vi "Send command (standalone).vi"(3 "Value":u16, 4 "Command":T2=17 items=["Measured main TEC temperature"=0, "Measured SHG heater temperature"=1, "Measured BRF heater temperature"=2, "Main TEC temperature command"=3, "SHG heater temperature command"=4, "BRF heater temperature command"=5, "Main TEC drive"=6, "SHG heater drive"=7, "BRF heater drive"=8, "Output power from photodiode"=9, "Output power setpoint (Get)"=10, "Output power setpoint (Set)"=11, "Start-up power setting (Get)"=12, "Start-up power setting (Set)"=13, "Measured LDD current"=14, "Maximum LDD current limit"=15, "16-bit fault code"=16, "Head serial number"=17, "Head board rev"=18, "Head type"=19, "LDD enable state"=20, "Key switch command (Get)"=24, "Key switch command (Set)"=25, "Key switch actual"=26, "Interlock status"=27, "Head hours"=28, "Photo or current mode command (Get)"=29, "Photo or current mode command (Set)"=30, "Photo or current mode actual"=31, "Analog input enable command (Get)"=32, "Analog input enable command (Set)"=33, "Analog input actual"=34, "Power supply glue input"=36, "Power supply glue output"=37], 5 "Selected laser":T1 items=["Green Laser", "Blue Laser"]) -> (0 "Error":errorcluster, 1 "response value":sgl, 2 "response":string)   [LabVIEW 2014]
uses:
  Commands.ctl
  Laser enum.ctl
  Coherent global.vi
panel:
  # "PN 06/11/2014"
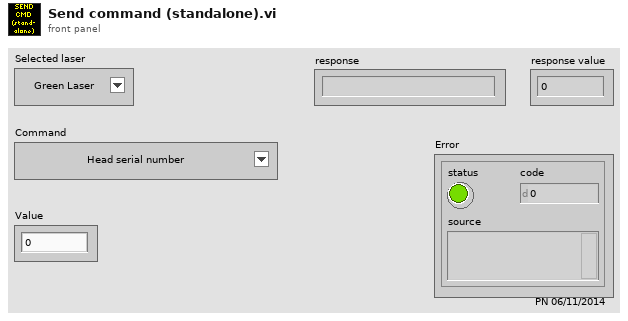
[diagram p1: front panel]
types:
  T1 = typedef "Laser enum.ctl" = u8
  T2 = typedef "Commands.ctl" = u8
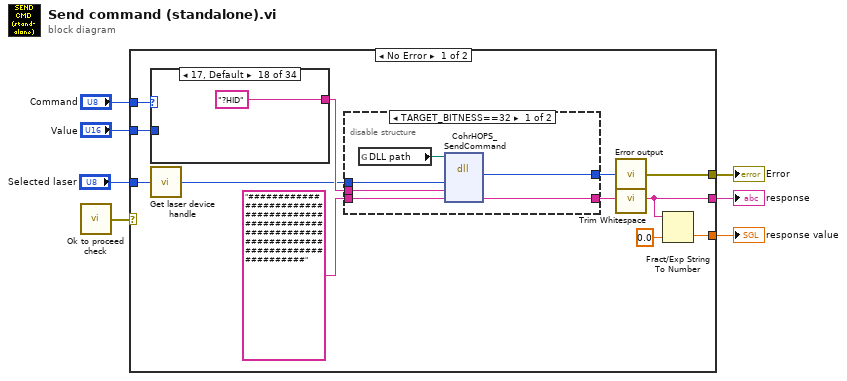
[diagram p0: block diagram]
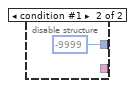
[diagram p2: hidden frame]
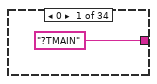
[diagram p3: hidden frame]
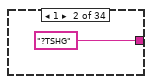
[diagram p4: hidden frame]
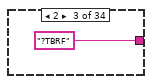
[diagram p5: hidden frame]
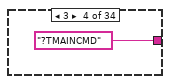
[diagram p6: hidden frame]
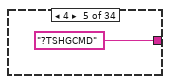
[diagram p7: hidden frame]
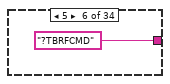
[diagram p8: hidden frame]
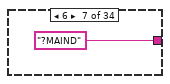
[diagram p9: hidden frame]
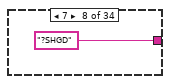
[diagram p10: hidden frame]
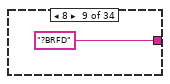
[diagram p11: hidden frame]
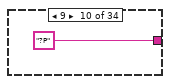
[diagram p12: hidden frame]
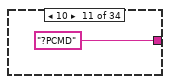
[diagram p13: hidden frame]
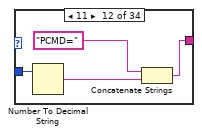
[diagram p14: hidden frame]
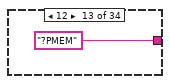
[diagram p15: hidden frame]
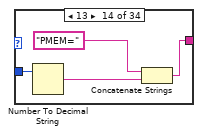
[diagram p16: hidden frame]
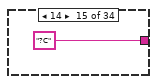
[diagram p17: hidden frame]
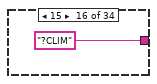
[diagram p18: hidden frame]
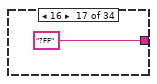
[diagram p19: hidden frame]
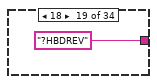
[diagram p20: hidden frame]
diagram:
  n1 = call "Ok to proceed check.vi"() -> ("Error"=w7:errorcluster)
  n2 = case shown="No Error" w7 {
    selector: w7 -> [_ w78]
    tunnel: [w14 sgl 0.0] -> w6
    tunnel: [w13 "" ("trimmed string")] -> w5
    tunnel: [w12 w78] -> w4
    tunnel: "Command" -> [w11 _]
    tunnel: "Value" -> [w10 _]
    tunnel: "Selected laser" -> [w9 _]
    frame No Error {
      n3 = case shown="17, Default" w11 {
        tunnel: ["?TMAIN" "?TSHG" "?TBRF" "?TMAINCMD" "?TSHGCMD" "?TBRFCMD" "?MAIND" "?SHGD" "?BRFD" "?P" "?PCMD" w38 "?PMEM" w43 "?C" "?CLIM" "?FF" "?HID" "?HBDREV" "?HTYPE" "?L" "?KSWCMD" w56 "?KSW" "?INT" "?HH" "?CMODECMD" w64 "?CMODE" "?ANACMD" w70 "?ANA" "?PSGLUEIN" "?PSGLUEOUT"] -> w18
        tunnel: w10 -> [_ _ _ _ _ _ _ _ _ _ _ w41 _ w46 _ _ _ _ _ _ _ _ w58 _ _ _ _ w66 _ _ w72 _ _ _]
        frame 0 {
        }
        frame 1 {
        }
        frame 2 {
        }
        frame 3 {
        }
        frame 4 {
        }
        frame 5 {
        }
        frame 6 {
        }
        frame 7 {
        }
        frame 8 {
        }
        frame 9 {
        }
        frame 10 {
        }
        frame 11 {
          n4 = Number To Decimal String(number=w41) -> (decimal integer string=w40:string)  [unwired: 1 in]
          n5 = Concatenate Strings("PCMD=", w40) -> (w38:string)
        }
        frame 12 {
        }
        frame 13 {
          n6 = Number To Decimal String(number=w46) -> (decimal integer string=w45:string)  [unwired: 1 in]
          n7 = Concatenate Strings("PMEM=", w45) -> (w43:string)
        }
        frame 14 {
        }
        frame 15 {
        }
        frame 16 {
        }
        frame 17, Default {
        }
        frame 18 {
        }
        frame 19 {
        }
        frame 20 {
        }
        frame 24 {
        }
        frame 25 {
          n8 = Number To Decimal String(number=w58) -> (decimal integer string=w55:string)  [unwired: 1 in]
          n9 = Concatenate Strings("KSWCMD=", w55) -> (w56:string)
        }
        frame 26 {
        }
        frame 27 {
        }
        frame 28 {
        }
        frame 29 {
        }
        frame 30 {
          n10 = Number To Decimal String(number=w66) -> (decimal integer string=w63:string)  [unwired: 1 in]
          n11 = Concatenate Strings("CMODECMD=", w63) -> (w64:string)
        }
        frame 31 {
        }
        frame 32 {
        }
        frame 33 {
          n12 = Number To Decimal String(number=w72) -> (decimal integer string=w69:string)  [unwired: 1 in]
          n13 = Concatenate Strings("ANACMD=", w69) -> (w70:string)
        }
        frame 34 {
        }
        frame 36 {
        }
        frame 37 {
        }
      }
      n14 = call "Get laser device handle.vi"("Selected laser"=w9) -> ("Device handle"=w8:u32)
      n15 = disable-structure shown="TARGET_BITNESS==32" {
        disable-tunnel: "####################################################################################################" ("headType") -> [w25 _]
        disable-tunnel: w8 -> [w24 _]
        disable-tunnel: w18 -> [w23 _]
        disable-tunnel: [w22 -9999 ("return value")] -> w17
        disable-tunnel: [w21 _] -> w16
        frame condition #0 (active) {
          n16 = global read "Coherent global.vi" "DLL path"() -> (w20:path)
          n17 = dll-call lib="C:/Program Files (x86)/Coherent/HOPS/CohrHOPS.dll" fn="CohrHOPS_SendCommand"(path in=w20, "handle"=w24, "command"=w23, "response"=w25) -> ("return value"=w22:i32, "response"=w21:string)  [unwired: 4 in, 2 out]
        }
        frame condition #1 {
        }
      }
      n18 = call "Error output.vi"("I32 err code"=w17) -> ("Error Out"=w12:errorcluster)
      n19 = call <vilib>:"Trim Whitespace.vi"("string"=w16) -> ("trimmed string"=w13:string)  [unwired: 1 in]
      n20 = Fract/Exp String To Number(string=w13, default (0 dbl)=sgl 0.0 ("default (0 DBL)")) -> (number=w14:sgl)  [unwired: 2 in, 1 out]
    }
    frame Error {
    }
  }
  "response" <- w5
  "response value" <- w6
  "Error" <- w4
